vi "Error Query.vi"(8 "error in (no error)":errorcluster, 11 "VISA resource name":refnum<visa-resource-name>) -> (0 "error out":errorcluster, 1 "Error Message":string, 2 "Error":i32, 3 "VISA resource name out":refnum<visa-resource-name>)   [LabVIEW 2014, in "Fluke 190 Series II.lvlib"]
doc: "Queries the error status of the Scopemeter's CPL interface.\nThe reply is a 16-bit word, presented as an integer value, in which each bit represents the Boolean value of a related error event."
uses:
  Fluke 190 Series II.lvlib
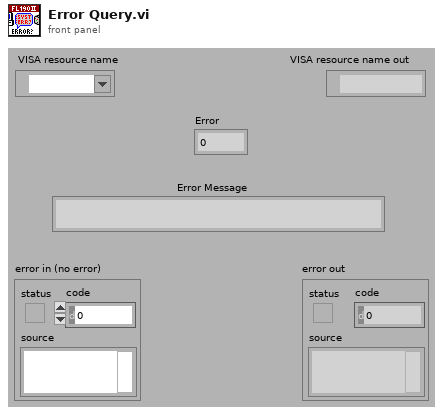
[diagram p1: front panel]
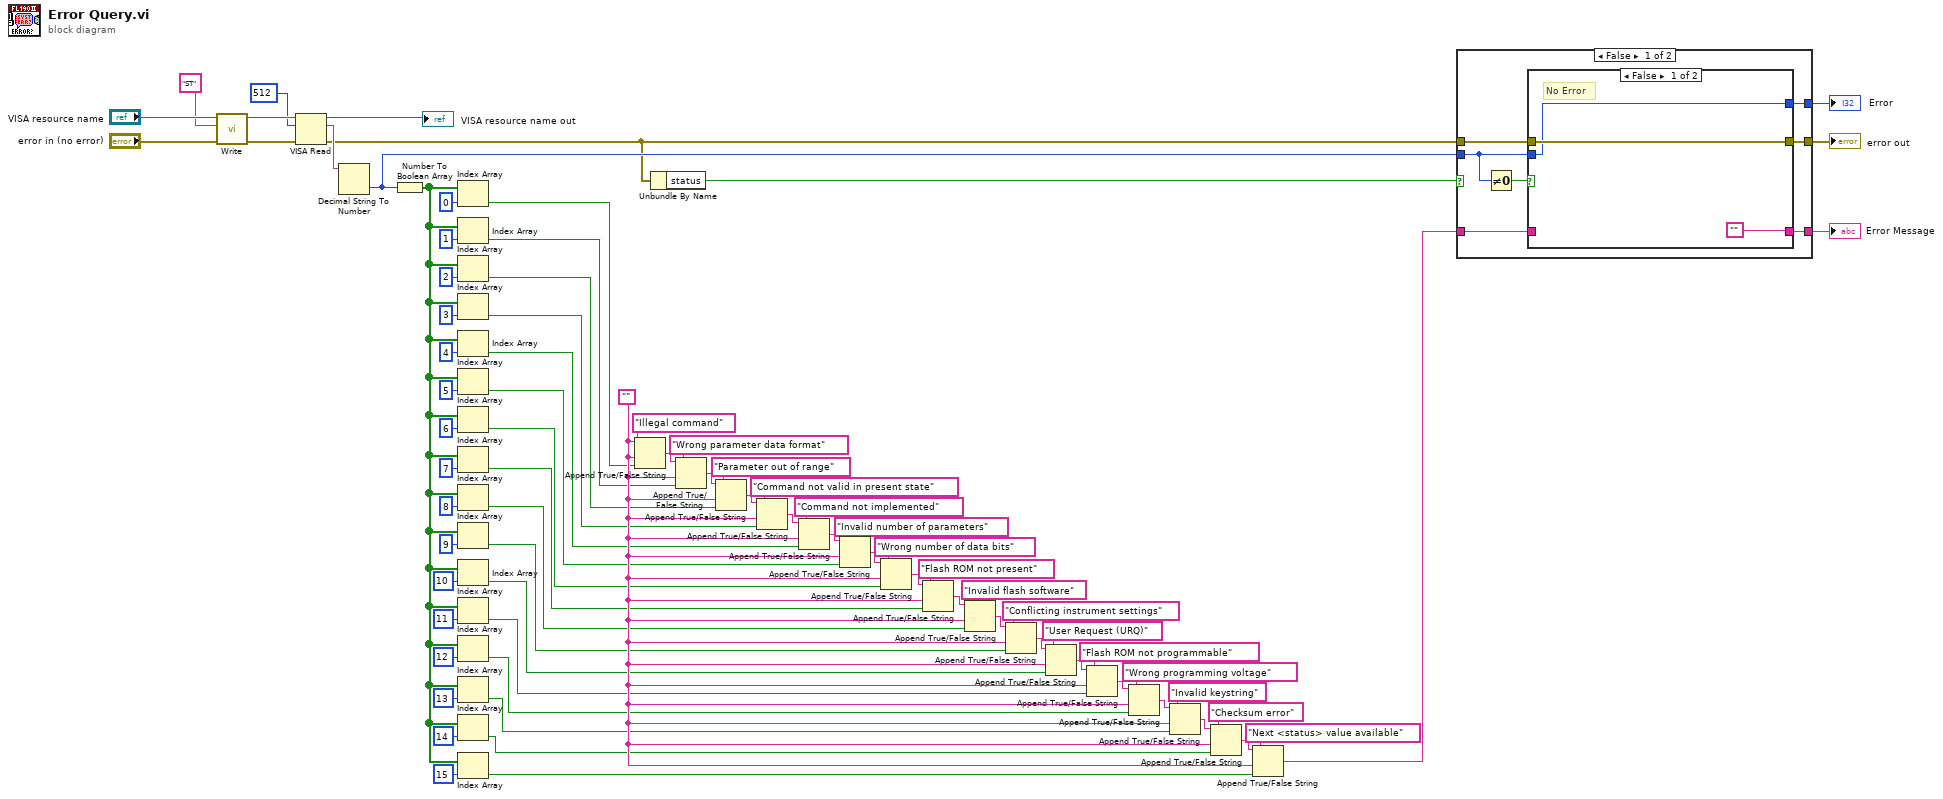
[diagram p0: block diagram]
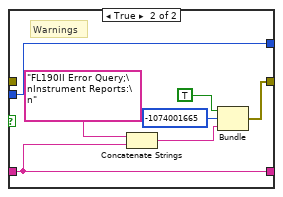
[diagram p2: hidden frame]
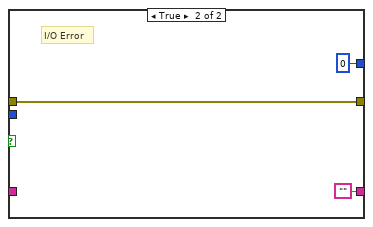
[diagram p3: hidden frame]
diagram:
  w34 = ""
  n1 = call "Write.vi"("error in (no error)"="error in (no error)", "Write Buffer"="ST", "VISA resource name"="VISA resource name") -> ("error out"=w76:errorcluster, "VISA resource name out"=w77:refnum<visa-resource-name>)  [unwired: 7 out]
  n2 = VISA Read(VISA resource name=w77, byte count=u32 512, error in (no error)=w76) -> (VISA resource name out=→"VISA resource name out":refnum<visa-resource-name>, read buffer=w73:string, error out=w52:errorcluster)  [unwired: 1 out]
  n3 = Decimal String To Number(string=w73) -> (number=w53:i32)  [unwired: 3 out]
  n4 = Number To Boolean Array(number=w53) -> (Boolean array=w56:bool[])
  n5 = Index Array(array=w56, index=0) -> (element=w2:bool)
  n6 = Index Array(array=w56, index=1) -> (element=w3:bool)
  n7 = Index Array(array=w56, index=2) -> (element=w4:bool)
  n8 = Index Array(array=w56, index=3) -> (element=w6:bool)
  n9 = Index Array(array=w56, index=4) -> (element=w7:bool)
  n10 = Index Array(array=w56, index=5) -> (element=w8:bool)
  n11 = Index Array(array=w56, index=6) -> (element=w5:bool)
  n12 = Index Array(array=w56, index=7) -> (element=w9:bool)
  n13 = Index Array(array=w56, index=8) -> (element=w10:bool)
  n14 = Index Array(array=w56, index=9) -> (element=w11:bool)
  n15 = Index Array(array=w56, index=10) -> (element=w12:bool)
  n16 = Index Array(array=w56, index=11) -> (element=w13:bool)
  n17 = Index Array(array=w56, index=12) -> (element=w14:bool)
  n18 = Index Array(array=w56, index=13) -> (element=w15:bool)
  n19 = Index Array(array=w56, index=14) -> (element=w16:bool)
  n20 = Index Array(array=w56, index=15) -> (element=w17:bool)
  n21 = Append True/False String(1:w2, 2:w34, 3:"Illegal command" ("true string"), 4:w34) -> (0:w49:string)
  n22 = Unbundle By Name(w52) -> ("status"=w51:bool)
  n23 = Append True/False String(1:w3, 2:w34, 3:"Wrong parameter data format" ("true string"), 4:w49) -> (0:w48:string)
  n24 = Append True/False String(1:w4, 2:w34, 3:"Parameter out of range" ("true string"), 4:w48) -> (0:w47:string)
  n25 = Append True/False String(1:w6, 2:w34, 3:"Command not valid in present state" ("true string"), 4:w47) -> (0:w46:string)
  n26 = Append True/False String(1:w7, 2:w34, 3:"Command not implemented" ("true string"), 4:w46) -> (0:w45:string)
  n27 = Append True/False String(1:w8, 2:w34, 3:"Invalid number of parameters" ("true string"), 4:w45) -> (0:w44:string)
  n28 = Append True/False String(1:w5, 2:w34, 3:"Wrong number of data bits" ("true string"), 4:w44) -> (0:w43:string)
  n29 = Append True/False String(1:w9, 2:w34, 3:"Flash ROM not present" ("true string"), 4:w43) -> (0:w35:string)
  n30 = Append True/False String(1:w10, 2:w34, 3:"Invalid flash software" ("true string"), 4:w35) -> (0:w42:string)
  n31 = Append True/False String(1:w11, 2:w34, 3:"Conflicting instrument settings" ("true string"), 4:w42) -> (0:w41:string)
  n32 = Append True/False String(1:w12, 2:w34, 3:"User Request (URQ)" ("true string"), 4:w41) -> (0:w40:string)
  n33 = Append True/False String(1:w13, 2:w34, 3:"Flash ROM not programmable" ("true string"), 4:w40) -> (0:w39:string)
  n34 = Append True/False String(1:w14, 2:w34, 3:"Wrong programming voltage" ("true string"), 4:w39) -> (0:w38:string)
  n35 = Append True/False String(1:w15, 2:w34, 3:"Invalid keystring" ("true string"), 4:w38) -> (0:w37:string)
  n36 = Append True/False String(1:w16, 2:w34, 3:"Checksum error" ("true string"), 4:w37) -> (0:w36:string)
  n37 = Append True/False String(1:w17, 2:w34, 3:"Next <status> value available" ("true string"), 4:w36) -> (0:w1:string)
  n38 = case shown="False" w51 {
    tunnel: w52 -> [w87 w100]
    tunnel: [w86 w100] -> w55
    tunnel: [w85 0] -> w50
    tunnel: [w84 ""] -> w54
    tunnel: w53 -> [w82 _]
    tunnel: w1 -> [w81 _]
    frame False {
      n39 = Not Equal To 0?(x=w82) -> (x != 0?=w83:bool)
      n40 = case shown="False" w83 {
        tunnel: [w90 w91] -> w86
        tunnel: w87 -> [w90 _]
        tunnel: w82 -> [w89 w97]
        tunnel: [w89 w97] -> w85
        tunnel: ["" w96] -> w84
        tunnel: w81 -> [_ w96]
        frame False {
          # "No Error"
        }
        frame True {
          # "Warnings"
          n41 = Concatenate Strings("FL190II Error Query;\nInstrument Reports:\n" ("string"), w96) -> (w94:string)
          n42 = Bundle(TRUE, -1074001665, w94) -> (w91:errorcluster)  [unwired: 1 out]
        }
      }
    }
    frame True {
      # "I/O Error"
    }
  }
  "error out" <- w55
  "Error Message" <- w54
  "Error" <- w50
